vi "Generate Data.vi"(4 "seed":i32=-1, 6 "sampling info":cluster{"Fs":dbl, "#s":dbl}={"Fs"=1000.0, "#s"=100.0}, 7 "reset":bool, 9 "noise (rms)":dbl, 10 "tones":T1(array[cluster])=[{"frequency"=21.0, "amplitude"=5.0, "phase"=0.0}, {"frequency"=20.0, "amplitude"=0.0, "phase"=0.0}] {"phase" format="%.2p"; "amplitude" format="%0.2p"; "frequency" format="%0.2p"}, 11 "signal":u16(ring) items=["uniform white", "uniform+uniform", "Gaussian white", "sine", "square"]) -> (2 "dt":dbl, 3 "Y":dbl[](array[numeric]))   [LabVIEW 2015]
uses:
  <vilib>/measure/NI_MABase.lvlib
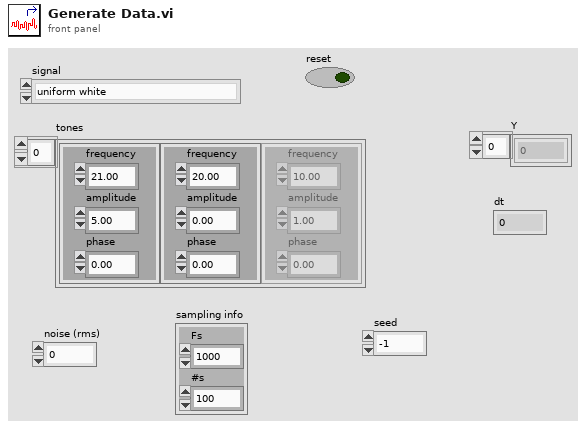
[diagram p1: front panel]
types:
  T1 = cluster{"frequency":dbl, "amplitude":dbl, "phase":dbl}[]
  T2 = enum16{"uniform white", "uniform+uniform", "Gaussian white", "sine", "square"}
  T3 = cluster{"frequency":dbl, "amplitude":dbl, "phase":dbl}
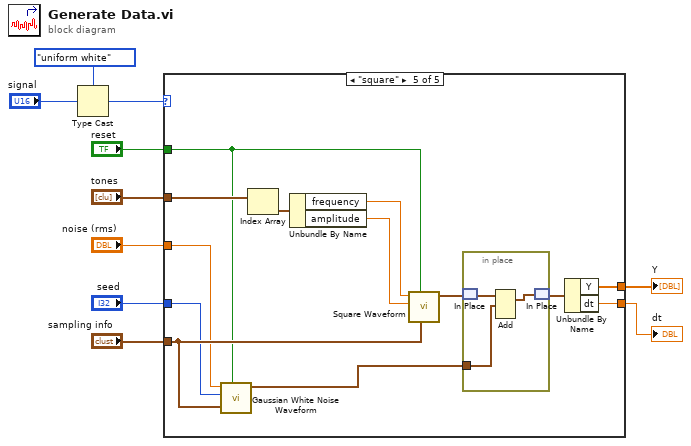
[diagram p0: block diagram]
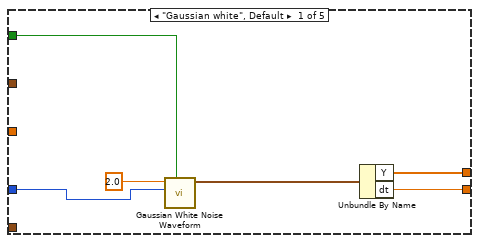
[diagram p2: hidden frame]
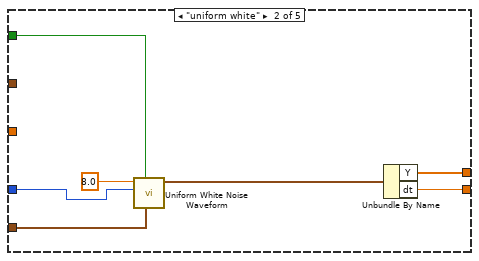
[diagram p3: hidden frame]
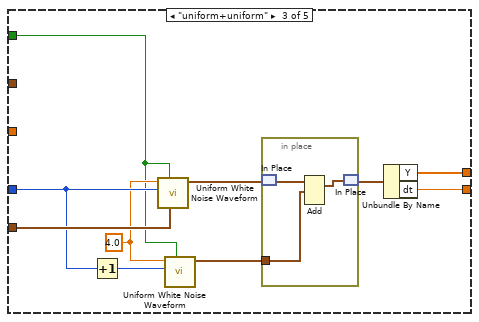
[diagram p4: hidden frame]
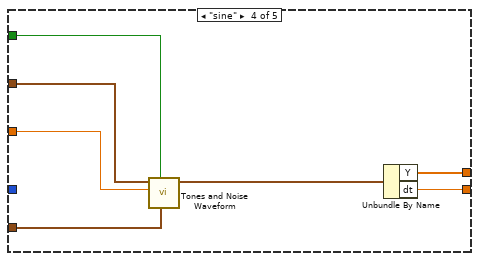
[diagram p5: hidden frame]
diagram:
  n1 = Type Cast(type=T2."uniform white" ("signal"), x="signal") -> (*(type *) &x=w1:T2)
  n2 = case shown="\"square\"" w1 {
    tunnel: "seed" -> [w16 w17 w28 _ w48]
    tunnel: [w13 w22 w33 w42 w56] -> w9
    tunnel: "reset" -> [w15 w21 w24 w41 w47]
    tunnel: "sampling info" -> [_ w20 w32 w40 w50]
    tunnel: "tones" -> [_ _ _ w39 w55]
    tunnel: "noise (rms)" -> [_ _ _ w38 w49]
    tunnel: [w12 w19 w31 w37 w45] -> w10
    frame "Gaussian white", Default {
      n3 = call <vilib>:"Gaussian White Noise Waveform.vi"("reset signal"=w15, "seed"=w16, "standard deviation"=2.0) -> ("signal out"=w14:waveform(dbl))  [unwired: 7 in, 1 out]
      n4 = Unbundle By Name(w14) -> ("Y"=w13:dbl[], "dt"=w12:dbl)
    }
    frame "uniform white" {
      n5 = call <vilib>:"Uniform White Noise Waveform.vi"("sampling info"=w20, "reset signal"=w21, "seed"=w17, "amplitude"=8.0) -> ("signal out"=w23:waveform(dbl))  [unwired: 6 in, 1 out]
      n6 = Unbundle By Name(w23) -> ("Y"=w22:dbl[], "dt"=w19:dbl)
    }
    frame "uniform+uniform" {
      w27 = 4.0 ("amplitude")
      n7 = Increment(x=w28) -> (x+1=w26:i32)
      n8 = call <vilib>:"Uniform White Noise Waveform.vi"("sampling info"=w32, "reset signal"=w24, "seed"=w28, "amplitude"=w27) -> ("signal out"=w30:waveform(dbl))  [unwired: 6 in, 1 out]
      n9 = call <vilib>:"Uniform White Noise Waveform.vi"("reset signal"=w24, "seed"=w26, "amplitude"=w27) -> ("signal out"=w25:waveform(dbl))  [unwired: 7 in, 1 out]
      n10 = in-place {
        in-place-border: w25 -> [w34]
        n11 = in-place-match #1(w30) -> (w36:waveform(dbl))
        n12 = Add(1:w34, 2:w36) -> (0:w35:waveform(dbl))  [unwired: 1 in, 1 out]
        n13 = in-place-match #1(w35) -> (w29:waveform(dbl))
      }
      n14 = Unbundle By Name(w29) -> ("Y"=w33:dbl[], "dt"=w31:dbl)
    }
    frame "sine" {
      n15 = call <vilib>:"Tones and Noise Waveform.vi"("sampling info"=w40, "reset signal"=w41, "noise (rms)"=w38, "tones"=w39) -> ("signal out"=w43:waveform(dbl))  [unwired: 6 in, 1 out]
      n16 = Unbundle By Name(w43) -> ("Y"=w42:dbl[], "dt"=w37:dbl)
    }
    frame "square" {
      n17 = call <vilib>:"Gaussian White Noise Waveform.vi"("sampling info"=w50, "reset signal"=w47, "seed"=w48, "standard deviation"=w49) -> ("signal out"=w46:waveform(dbl))  [unwired: 6 in, 1 out]
      n18 = Index Array(array=w55) -> (element=w54:T3)  [unwired: 1 in]
      n19 = Unbundle By Name(w54) -> ("frequency"=w53:dbl, "amplitude"=w52:dbl)
      n20 = call <vilib>:"Square Waveform.vi"("sampling info"=w50, "reset signal"=w47, "amplitude"=w52, "frequency"=w53) -> ("signal out"=w51:waveform(dbl))  [unwired: 6 in, 1 out]
      n21 = in-place {
        in-place-border: w46 -> [w58]
        n22 = in-place-match #2(w51) -> (w59:waveform(dbl))
        n23 = Add(1:w58, 2:w59) -> (0:w57:waveform(dbl))  [unwired: 1 in, 1 out]
        n24 = in-place-match #2(w57) -> (w44:waveform(dbl))
      }
      n25 = Unbundle By Name(w44) -> ("Y"=w56:dbl[], "dt"=w45:dbl)
    }
  }
  "dt" <- w10
  "Y" <- w9
